vi "EmergencyStop_Main.vi"() -> ()   [LabVIEW 2014]
uses:
  TowerLight_class/TrafficLight.ctl
  EmergencyController_class/EmergencyController.lvclass
  XmlLogger_class/XmlLogger.lvclass
  TowerLight_class/TowerLight.lvclass
  ConveyorBelt_class/ConveyorBelt.lvclass
  IDisposable_Interface/IDisposable.lvclass
panel:
  out "E-Time Time":u32 caption="ms"
  out "Time to Stop":u32 caption="ms"
  out "LogString":string
  out "TowerLight":T1
  out "error out":errorcluster
  in  "Stop":bool
  in  "Emergency":bool
  out "Slide":u8(slide) scale=0.0..100.0
  # "Press E-Stop to\nsignal to all subscribed objects\nthat they should have to handle an Emergency Stop."
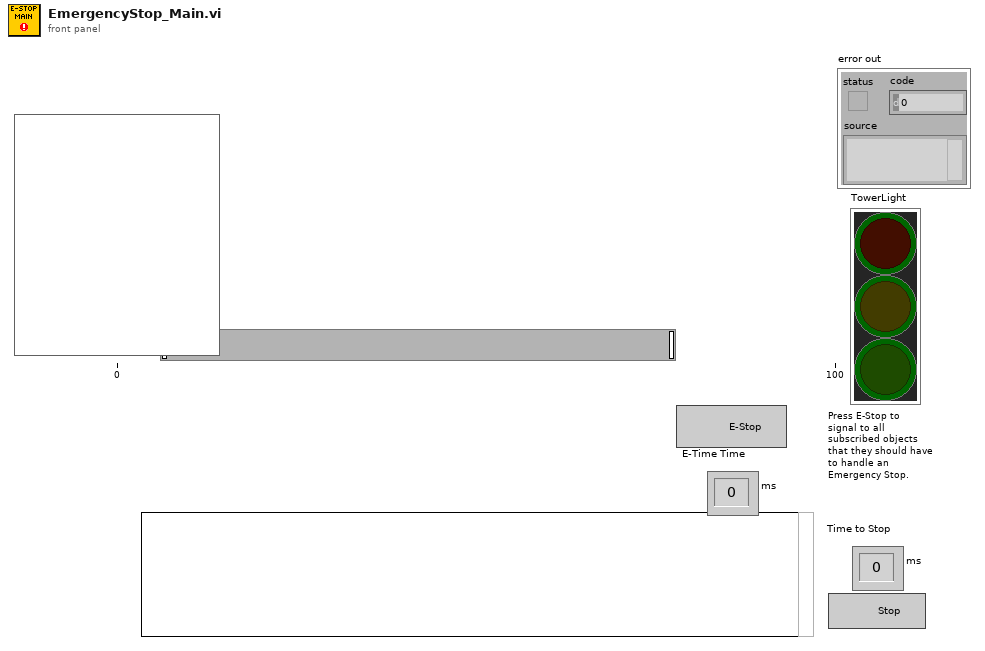
[diagram p1: front panel]
types:
  T1 = typedef "TowerLight.lvclass/TrafficLight.ctl" = cluster{"Red":bool, "Yellow":bool, "Green":bool}
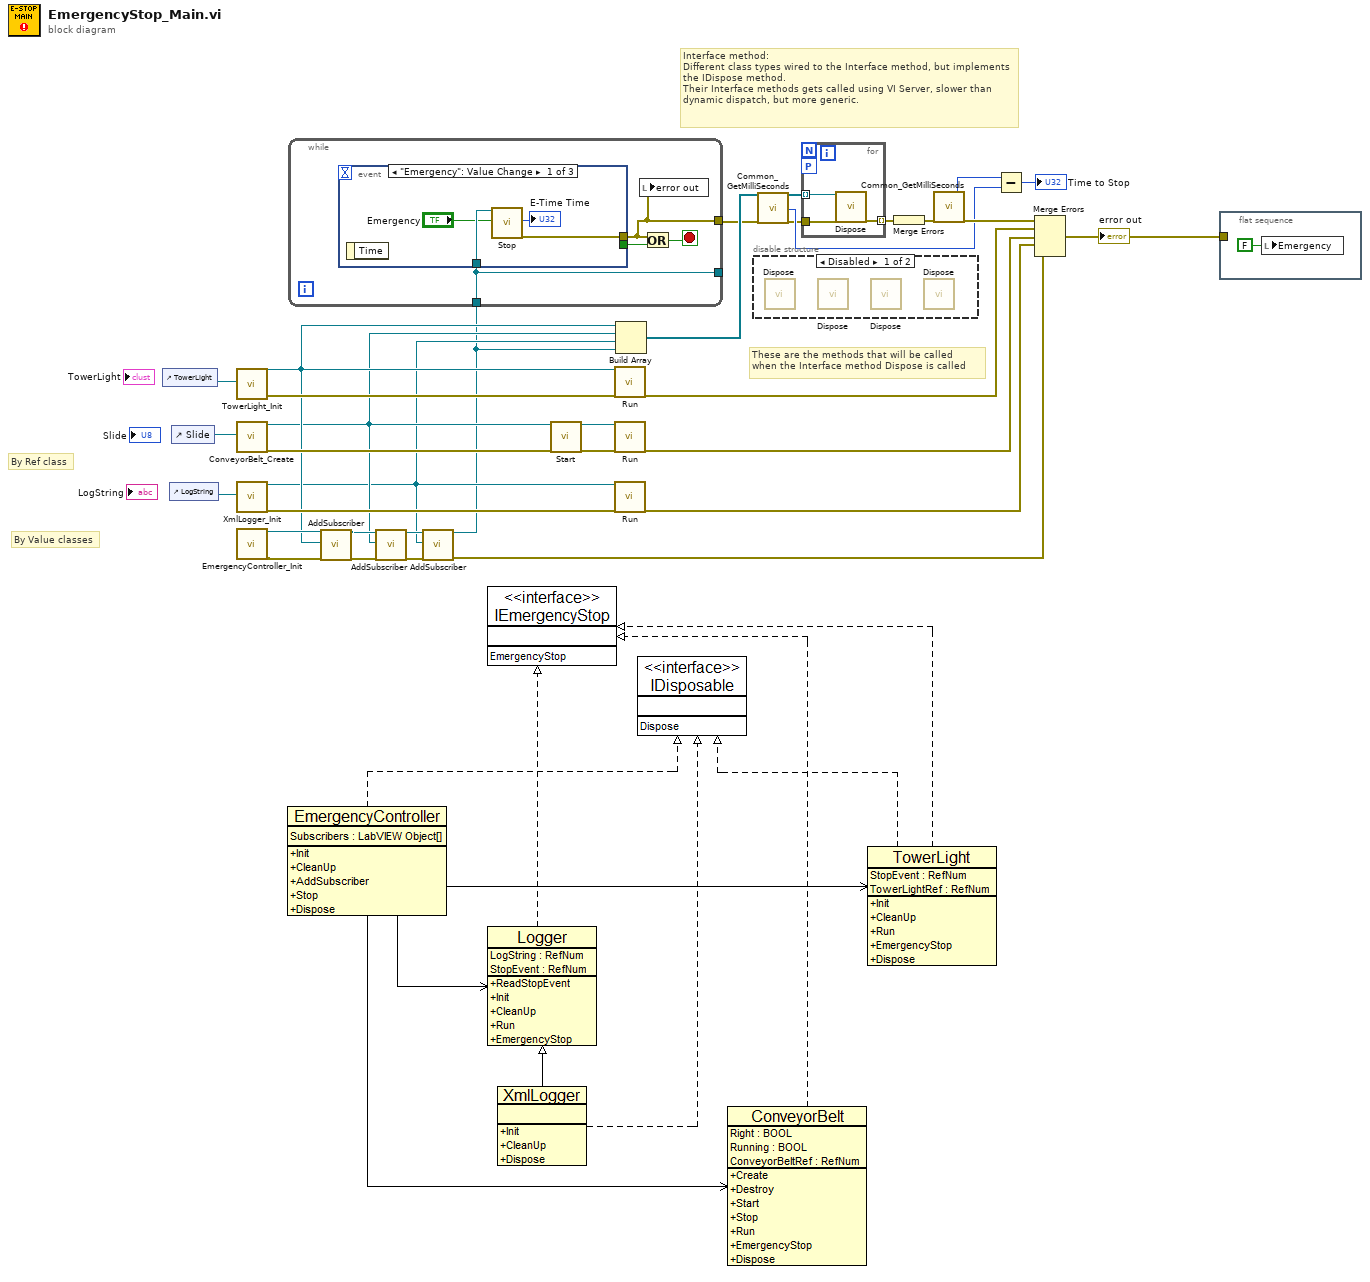
[diagram p0: block diagram]
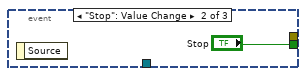
[diagram p3: hidden frame]
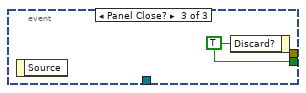
[diagram p4: hidden frame]
diagram:
  # "By Ref class"
  # "By Value classes"
  # "By Value classes"
  # "By Value classes"
  # "These are the methods that will be called\nwhen the Interface method Dispose is called"
  # "Interface method:\nDifferent class types wired to the Interface method, but implements the IDispose method.\nTheir Interface methods gets called using VI Server, slower than dynamic dispatch, but more generic."
  n1 = control-ref of="TowerLight"() -> (w27:refnum<vi>)
  n2 = control-ref of="LogString"() -> (w21:refnum<vi>)
  n3 = control-ref of="Slide"() -> (w32:refnum<vi>)
  n4 = call "TowerLight_Init.vi"("TowerLightRef"=w27) -> ("object out"=w15:refnum<class "TowerLight.lvclass">, "error out"=w26:errorcluster)  [unwired: 17 in]
  n5 = call "ConveyorBelt_Create.vi"("ConveyorBeltRef"=w32) -> ("reference out"=w14:refnum<class "ConveyorBelt.lvclass">, "error out"=w31:errorcluster)  [unwired: 17 in]
  n6 = call "XmlLogger_Init.vi"("LogString"=w21) -> ("object out"=w13:refnum<class "XmlLogger.lvclass">, "error out"=w18:errorcluster)  [unwired: 17 in]
  n7 = call "EmergencyController_Init.vi"() -> ("object out"=w29:refnum<class "EmergencyController.lvclass">, "error out"=w28:errorcluster)  [unwired: 18 in]
  n8 = call-dynamic "AddSubscriber.vi"("object in"=w29, "EmergancyStopObject"=w15, "error in (no error)"=w28) -> ("object out"=w25:refnum<class "EmergencyController.lvclass">, "error out"=w24:errorcluster)  [unwired: 15 in]
  n9 = call-dynamic "AddSubscriber.vi"("object in"=w25, "EmergancyStopObject"=w14, "error in (no error)"=w24) -> ("object out"=w20:refnum<class "EmergencyController.lvclass">, "error out"=w19:errorcluster)  [unwired: 15 in]
  n10 = call-dynamic "AddSubscriber.vi"("object in"=w20, "EmergancyStopObject"=w13, "error in (no error)"=w19) -> ("object out"=w12:refnum<class "EmergencyController.lvclass">, "error out"=w10:errorcluster)  [unwired: 15 in]
  n11 = while {
    tunnel: w12 -> [w34]
    tunnel: [w34] -> _
    tunnel: [w33] -> w6
    stop <- w35 stop-if-true
    n12 = event shown="[0] \"Emergency\": Value Change" {
      selector: _ -> [_ _ _]
      dyn-events: _ -> [_ _ _]
      timeout: _ -> [_ _ _]
      tunnel: [w38 _ _] -> w33
      tunnel: w34 -> [w40 _ _]
      tunnel: [_ "Stop" w42] -> w36
      event "Emergency": Value Change {
        n13 = event-data() -> ()  [unwired: 1 in, 1 out]
        n14 = call-dynamic "Stop.vi"("object in"=w40, "Emergancy"="Emergency") -> ("Time(ms)"=→"E-Time Time":u32, "error out"=w38:errorcluster)  [unwired: 15 in, 1 out]
      }
      event "Stop": Value Change {
        n15 = event-data() -> ()  [unwired: 1 in, 1 out]
      }
      event Panel Close? {
        w42 = TRUE ("Discard?")
        n16 = event-data() -> ()  [unwired: 1 in, 1 out]
        n17 = event-data("Discard?"=w42) -> ()  [unwired: 1 in, 1 out]
      }
    }
    n18 = local write "error out"(w33) -> ()
    n19 = Or(x=w33, y=w36) -> (x .or. y?=w35:bool)
  }
  n20 = call-dynamic "Start.vi"("reference in"=w14, "error in (no error)"=w31) -> ("reference out"=w23:refnum<class "ConveyorBelt.lvclass">, "error out"=w30:errorcluster)  [unwired: 16 in]
  n21 = call-dynamic "Run.vi"("object in"=w15, "error in (no error)"=w26) -> ("error out"=w17:errorcluster)  [unwired: 16 in, 1 out]
  n22 = call-dynamic "Run.vi"("reference in"=w23, "error in (no error)"=w30) -> ("error out"=w16:errorcluster)  [unwired: 16 in, 1 out]
  n23 = call-dynamic "Run.vi"("object in"=w13, "error in (no error)"=w18) -> ("error out"=w11:errorcluster)  [unwired: 16 in, 1 out]
  n24 = Build Array(w15, w14, w13, w12) -> (w22:refnum<class>[])
  n25 = disable-structure shown="Disabled" {
    frame Disabled {
      n26 = call-dynamic "Dispose.vi"() -> ()  [unwired: 18 in, 2 out]
      n27 = call-dynamic "Dispose.vi"() -> ()  [unwired: 18 in, 2 out]
      n28 = call-dynamic "Dispose.vi"() -> ()  [unwired: 18 in, 2 out]
      n29 = call-dynamic "Dispose.vi"() -> ()  [unwired: 18 in, 2 out]
    }
    frame Enabled {
    }
  }
  n30 = call "Common_GetMilliSeconds.vi"("error in (no error)"=w6) -> ("msValue"=w4:u32, "error out"=w3:errorcluster)  [unwired: 17 in]
  n31 = for {
    tunnel: w22 -> [w45] mode=indexing
    tunnel: w3 -> [w44]
    tunnel: [w43] -> w2 mode=indexing
    workers-P: _ -> [_]
    n32 = call "Dispose.vi"("Interface In"=w45, "error in (no error)"=w44) -> ("error out"=w43:errorcluster)  [unwired: 16 in, 1 out]
  }
  n33 = Merge Errors(w2) -> (w1:errorcluster)
  n34 = call "Common_GetMilliSeconds.vi"("error in (no error)"=w1) -> ("msValue"=w7:u32, "error out"=w5:errorcluster)  [unwired: 17 in]
  n35 = Subtract(x=w7, y=w4) -> (x-y=→"Time to Stop":u32)
  n36 = Merge Errors(w5, w17, w16, w11, w10) -> (w9:errorcluster)
  "error out" <- w9
  n37 = flat-sequence {
    tunnel: w9 -> [_]
    frame #0 {
      n38 = local write "Emergency"(FALSE ("Emergency")) -> ()
    }
  }
